vi "Pressure Regulator.vi"(7 "Indicators":T2, 8 "error in":errorcluster, 10 "Pressure Controller Port":refnum<visa-resource-name>="COM1", 11 "Controls":T1) -> (0 "error out":errorcluster)   [LabVIEW 2012, in "Pressure Regulator Controller.lvlib"]
uses:
  Pressure Regulator Controller.lvlib
  <vilib>/Instr/_visa.llb/VISA Configure Serial Port (Serial Instr).vi
panel:
  out "read buffer":string
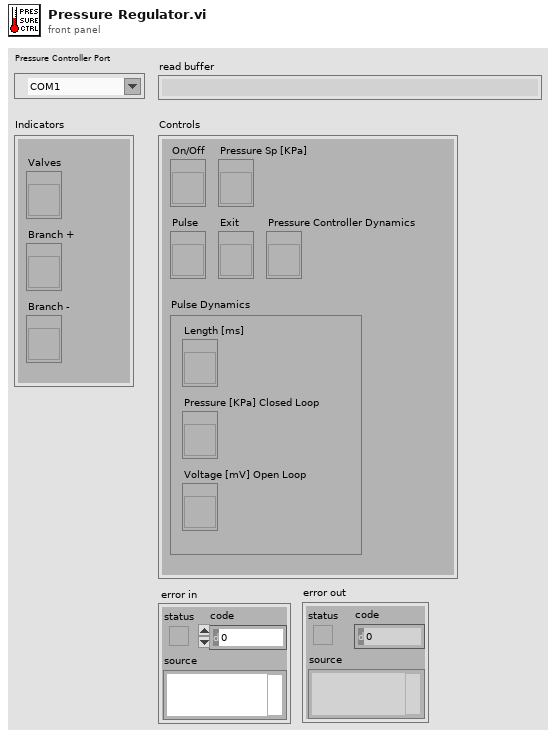
[diagram p1: front panel]
types:
  T1 = cluster{"Pulse Dynamics":cluster{"Length [ms]":refnum<vi>, "Pressure [KPa] Closed Loop":refnum<vi>, "Voltage [mV] Open Loop":refnum<vi>}, "On/Off":refnum<vi>, "Exit":refnum<vi>, "Pulse":refnum<vi>, "Pressure Sp [KPa]":refnum<vi>, "Pressure Controller Dynamics":refnum<vi>}
  T2 = cluster{"Valves":refnum<vi>, "Branch +":refnum<vi>, "Branch -":refnum<vi>}
  T3 = cluster{"Positive Branch":cluster{"Kp":dbl, "Ki":dbl, "Kd":dbl}, "Negative Branch":cluster{"Kp":dbl, "Ki":dbl, "Kd":dbl}}
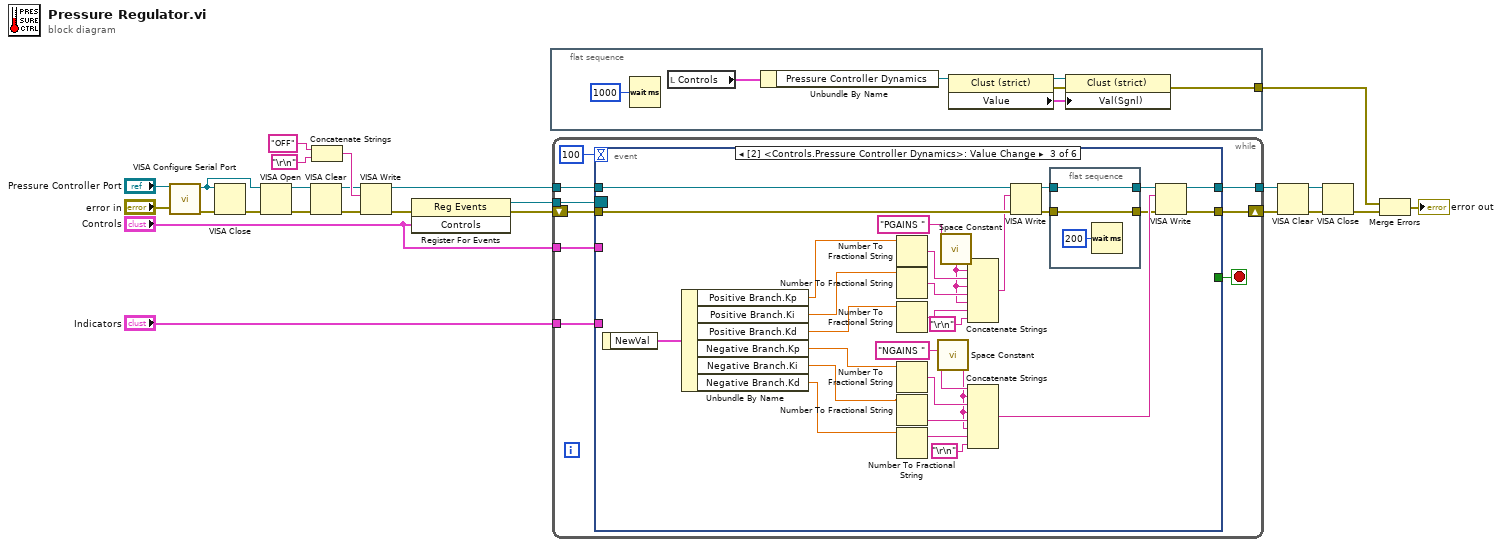
[diagram p0: block diagram]
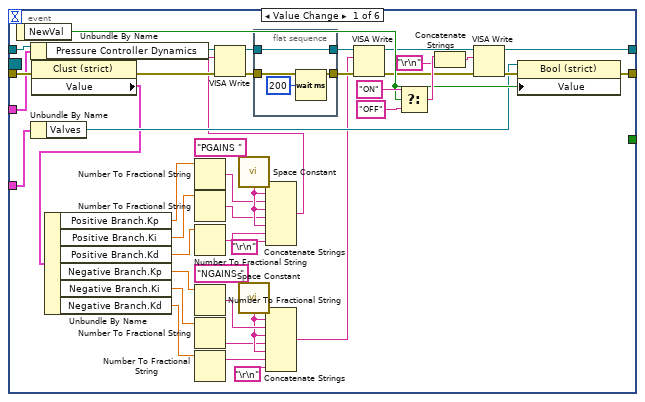
[diagram p2: hidden frame]
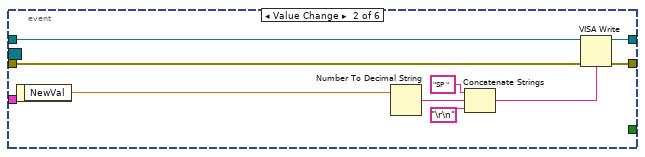
[diagram p3: hidden frame]
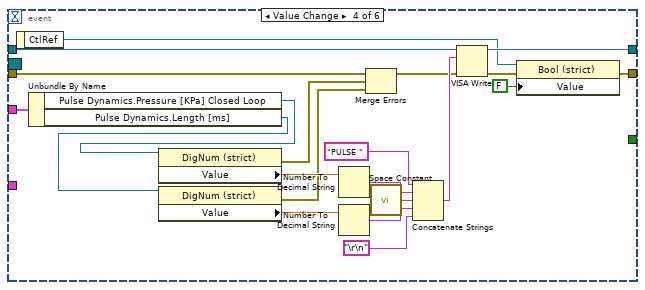
[diagram p4: hidden frame]
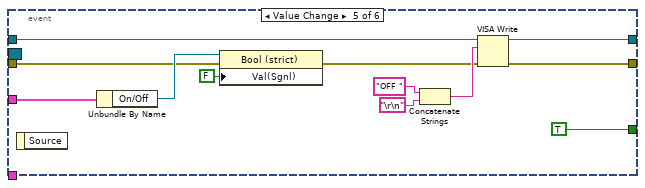
[diagram p5: hidden frame]
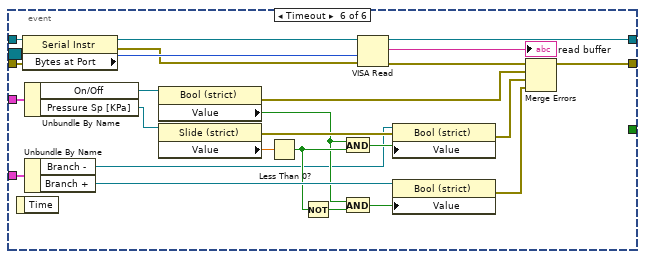
[diagram p6: hidden frame]
diagram:
  n1 = call-poly "VISA Configure Serial Port"("VISA resource name"="Pressure Controller Port", "error in (no error)"="error in") -> ("VISA resource name out"=w1:refnum<visa-resource-name>, "error out"=w3:errorcluster)  [unwired: 12 in]
  n2 = VISA Close(VISA resource name=w1, error in (no error)=w3) -> (error out=w2:errorcluster)
  n3 = VISA Open(error in (no error)=w2, VISA resource name=w1) -> (VISA resource name=w16:refnum<visa-resource-name>, error out=w17:errorcluster)  [unwired: 3 in]
  n4 = VISA Clear(VISA resource name=w16, error in (no error)=w17) -> (VISA resource name out=w10:refnum<visa-resource-name>, error out=w11:errorcluster)
  n5 = Concatenate Strings("OFF" ("string"), "\r\n") -> (w13:string)
  n6 = VISA Write(VISA resource name=w10, write buffer=w13, error in (no error)=w11) -> (VISA resource name out=w9:refnum<visa-resource-name>, error out=w12:errorcluster)  [unwired: 1 out]
  n7 = register-events(error in=w12, "Controls") -> (reference out=w19:refnum<event-registration>, error out=w21:errorcluster)  [unwired: 1 in]
  n8 = flat-sequence {
    tunnel: [w26] -> w6
    frame #0 {
      n9 = Wait (ms)(milliseconds to wait=u32 1000) -> ()  [unwired: 1 out]
      n10 = local read "Controls"() -> (w32:T1)
      n11 = Unbundle By Name(w32) -> ("Pressure Controller Dynamics"=w28:refnum<vi>)
      n12 = property class="Clust (strict)"(reference=w28) -> (reference out=w31:refnum<vi>, error out=w30:errorcluster, "Value"=w29:T3)  [unwired: 1 in]
      n13 = property class="Clust (strict)"(reference=w31, error in=w30, "Val(Sgnl)"=w29) -> (error out=w26:errorcluster)  [unwired: 1 out]
    }
  }
  n14 = while {
    tunnel: w9 -> [w33]
    shift-right: [w41] -> w23
    shift-left: w21 -> [w34]
    tunnel: [w39] -> w22
    tunnel: "Indicators" -> [w38]
    tunnel: "Controls" -> [w37]
    tunnel: w19 -> [w36]
    stop <- w35 stop-if-true
    n15 = event shown="[2] <Controls.Pressure Controller Dynamics>: Value Change" {
      selector: w36 -> [_ _ _ _ _ _]
      dyn-events: _ -> [_ _ _ _ _ _]
      timeout: 100 -> [_ _ _ _ _ _]
      tunnel: w33 -> [w46 w88 w125 w148 w159 w183]
      tunnel: [w76 w96 w118 w143 w161 w176] -> w41
      tunnel: w34 -> [w73 w89 w124 w135 w150 w181]
      tunnel: [w84 w95 w119 w149 w160 w182] -> w39
      tunnel: w38 -> [w78 _ _ _ _ w175]
      tunnel: w37 -> [w72 _ _ w140 w153 w174]
      tunnel: [_ _ _ _ TRUE _] -> w35
      event Value Change {
        n16 = event-data() -> ("NewVal"=w75:bool)  [unwired: 1 in]
        n17 = Unbundle By Name(w72) -> ("Pressure Controller Dynamics"=w71:refnum<vi>)
        n18 = Unbundle By Name(w78) -> ("Valves"=w74:refnum<vi>)
        n19 = property class="Clust (strict)"(reference=w71, error in=w73) -> (error out=w47:errorcluster, "Value"=w52:T3)  [unwired: 1 out]
        n20 = Unbundle By Name(w52) -> ("Positive Branch.Kp"=w62:dbl, "Positive Branch.Ki"=w61:dbl, "Positive Branch.Kd"=w60:dbl, "Negative Branch.Kp"=w67:dbl, "Negative Branch.Ki"=w54:dbl, "Negative Branch.Kd"=w66:dbl)
        n21 = Number To Fractional String(number=w62) -> (F-format string=w65:string)  [unwired: 3 in]
        n22 = Number To Fractional String(number=w61) -> (F-format string=w63:string)  [unwired: 3 in]
        n23 = Number To Fractional String(number=w60) -> (F-format string=w64:string)  [unwired: 3 in]
        n24 = Number To Fractional String(number=w67) -> (F-format string=w59:string)  [unwired: 3 in]
        n25 = Number To Fractional String(number=w54) -> (F-format string=w53:string)  [unwired: 3 in]
        n26 = Number To Fractional String(number=w66) -> (F-format string=w58:string)  [unwired: 3 in]
        n27 = call <vilib>:"Space Constant.vi"() -> ("String"=w69:string)
        n28 = call <vilib>:"Space Constant.vi"() -> ("String"=w56:string)
        n29 = flat-sequence {
          tunnel: [w87] -> w51
          tunnel: w50 -> [w87]
          tunnel: [w86] -> w49
          tunnel: w48 -> [w86]
          frame #0 {
            n30 = Wait (ms)(milliseconds to wait=u32 200) -> ()  [unwired: 1 out]
          }
        }
        n31 = Concatenate Strings("PGAINS " ("string"), w69, w65, w69, w63, w69, w64, "\r\n") -> (w45:string)
        n32 = VISA Write(VISA resource name=w46, write buffer=w45, error in (no error)=w47) -> (VISA resource name out=w50:refnum<visa-resource-name>, error out=w48:errorcluster)  [unwired: 1 out]
        n33 = Concatenate Strings("NGAINS " ("string"), w56, w59, w56, w53, w56, w58, "\r\n") -> (w44:string)
        n34 = VISA Write(VISA resource name=w51, write buffer=w44, error in (no error)=w49) -> (VISA resource name out=w43:refnum<visa-resource-name>, error out=w42:errorcluster)  [unwired: 1 out]
        n35 = Select(t="ON" ("string"), s=w75, f="OFF") -> (s? t:f=w80:string)
        n36 = Concatenate Strings(w80, "\r\n") -> (w83:string)
        n37 = VISA Write(VISA resource name=w43, write buffer=w83, error in (no error)=w42) -> (VISA resource name out=w84:refnum<visa-resource-name>, error out=w77:errorcluster)  [unwired: 1 out]
        n38 = property class="Bool (strict)"(reference=w74, error in=w77, "Value"=w75) -> (error out=w76:errorcluster)  [unwired: 1 out]
      }
      event Value Change {
        n39 = event-data() -> ("NewVal"=w91:dbl)  [unwired: 1 in]
        n40 = Number To Decimal String(number=w91) -> (decimal integer string=w90:string)  [unwired: 1 in]
        n41 = Concatenate Strings("SP " ("string"), w90, "\r\n") -> (w94:string)
        n42 = VISA Write(VISA resource name=w88, write buffer=w94, error in (no error)=w89) -> (VISA resource name out=w95:refnum<visa-resource-name>, error out=w96:errorcluster)  [unwired: 1 out]
      }
      event Value Change {
        n43 = event-data() -> ("NewVal"=w123:T3)  [unwired: 1 in]
        n44 = Unbundle By Name(w123) -> ("Positive Branch.Kp"=w110:dbl, "Positive Branch.Ki"=w109:dbl, "Positive Branch.Kd"=w108:dbl, "Negative Branch.Kp"=w121:dbl, "Negative Branch.Ki"=w104:dbl, "Negative Branch.Kd"=w120:dbl)
        n45 = Number To Fractional String(number=w110) -> (F-format string=w102:string)  [unwired: 3 in]
        n46 = Number To Fractional String(number=w109) -> (F-format string=w111:string)  [unwired: 3 in]
        n47 = Number To Fractional String(number=w108) -> (F-format string=w112:string)  [unwired: 3 in]
        n48 = Number To Fractional String(number=w121) -> (F-format string=w107:string)  [unwired: 3 in]
        n49 = Number To Fractional String(number=w104) -> (F-format string=w103:string)  [unwired: 3 in]
        n50 = Number To Fractional String(number=w120) -> (F-format string=w106:string)  [unwired: 3 in]
        n51 = call <vilib>:"Space Constant.vi"() -> ("String"=w98:string)
        n52 = call <vilib>:"Space Constant.vi"() -> ("String"=w101:string)
        n53 = Concatenate Strings("PGAINS " ("string"), w101, w102, w101, w111, w101, w112, "\r\n") -> (w97:string)
        n54 = Concatenate Strings("NGAINS " ("string"), w98, w107, w98, w103, w98, w106, "\r\n") -> (w117:string)
        n55 = VISA Write(VISA resource name=w125, write buffer=w97, error in (no error)=w124) -> (VISA resource name out=w115:refnum<visa-resource-name>, error out=w113:errorcluster)  [unwired: 1 out]
        n56 = flat-sequence {
          tunnel: [w128] -> w116
          tunnel: w115 -> [w128]
          tunnel: [w127] -> w114
          tunnel: w113 -> [w127]
          frame #0 {
            n57 = Wait (ms)(milliseconds to wait=u32 200) -> ()  [unwired: 1 out]
          }
        }
        n58 = VISA Write(VISA resource name=w116, write buffer=w117, error in (no error)=w114) -> (VISA resource name out=w119:refnum<visa-resource-name>, error out=w118:errorcluster)  [unwired: 1 out]
      }
      event Value Change {
        n59 = event-data() -> ("CtlRef"=w142:refnum<vi>)  [unwired: 1 in]
        n60 = Unbundle By Name(w140) -> ("Pulse Dynamics.Pressure [KPa] Closed Loop"=w139:refnum<vi>, "Pulse Dynamics.Length [ms]"=w138:refnum<vi>)
        n61 = property class="DigNum (strict)"(reference=w139) -> (error out=w133:errorcluster, "Value"=w137:dbl)  [unwired: 1 in, 1 out]
        n62 = property class="DigNum (strict)"(reference=w138) -> (error out=w132:errorcluster, "Value"=w136:dbl)  [unwired: 1 in, 1 out]
        n63 = Number To Decimal String(number=w137) -> (decimal integer string=w145:string)  [unwired: 1 in]
        n64 = Number To Decimal String(number=w136) -> (decimal integer string=w131:string)  [unwired: 1 in]
        n65 = Merge Errors(w135, w133, w132) -> (w134:errorcluster)
        n66 = call <vilib>:"Space Constant.vi"() -> ("String"=w129:string)
        n67 = Concatenate Strings("PULSE " ("string"), w145, w129, w131, "\r\n") -> (w147:string)
        n68 = VISA Write(VISA resource name=w148, write buffer=w147, error in (no error)=w134) -> (VISA resource name out=w149:refnum<visa-resource-name>, error out=w144:errorcluster)  [unwired: 1 out]
        n69 = property class="Bool (strict)"(reference=w142, error in=w144, "Value"=FALSE) -> (error out=w143:errorcluster)  [unwired: 1 out]
      }
      event Value Change {
        n70 = event-data() -> ()  [unwired: 1 in, 1 out]
        n71 = Unbundle By Name(w153) -> ("On/Off"=w152:refnum<vi>)
        n72 = property class="Bool (strict)"(reference=w152, error in=w150, "Val(Sgnl)"=FALSE ("Value")) -> (error out=w151:errorcluster)  [unwired: 1 out]
        n73 = Concatenate Strings("OFF " ("string"), "\r\n") -> (w158:string)
        n74 = VISA Write(VISA resource name=w159, write buffer=w158, error in (no error)=w151) -> (VISA resource name out=w160:refnum<visa-resource-name>, error out=w161:errorcluster)  [unwired: 1 out]
      }
      event Timeout {
        n75 = event-data() -> ()  [unwired: 1 in, 1 out]
        n76 = property class="Serial Instr"(reference=w183, error in=w181) -> (reference out=w186:refnum<visa-resource-name>, error out=w184:errorcluster, "Bytes at Port"=w185:u32)
        n77 = Unbundle By Name(w174) -> ("On/Off"=w171:refnum<vi>, "Pressure Sp [KPa]"=w172:refnum<vi>)
        n78 = Unbundle By Name(w175) -> ("Branch -"=w165:refnum<vi>, "Branch +"=w177:refnum<vi>)
        n79 = property class="Bool (strict)"(reference=w171) -> (error out=w164:errorcluster, "Value"=w167:bool)  [unwired: 1 in, 1 out]
        n80 = property class="Slide (strict)"(reference=w172) -> (error out=w169:errorcluster, "Value"=w170:dbl)  [unwired: 1 in, 1 out]
        n81 = Less Than 0?(x=w170) -> (x < 0?=w168:bool)
        n82 = Not(x=w168) -> (.not. x?=w166:bool)
        n83 = And(x=w167, y=w168) -> (x .and. y?=w178:bool)
        n84 = And(x=w167, y=w166) -> (x .and. y?=w179:bool)
        n85 = VISA Read(VISA resource name=w186, byte count=w185, error in (no error)=w184) -> (VISA resource name out=w182:refnum<visa-resource-name>, read buffer=→"read buffer":string, error out=w173:errorcluster)  [unwired: 1 out]
        n86 = property class="Bool (strict)"(reference=w165, error in=w169, "Value"=w178) -> (error out=w163:errorcluster)  [unwired: 1 out]
        n87 = property class="Bool (strict)"(reference=w177, "Value"=w179) -> (error out=w162:errorcluster)  [unwired: 1 in, 1 out]
        n88 = Merge Errors(w173, w164, w163, w162) -> (w176:errorcluster)
      }
    }
  }
  n89 = VISA Clear(VISA resource name=w22, error in (no error)=w23) -> (VISA resource name out=w25:refnum<visa-resource-name>, error out=w24:errorcluster)
  n90 = VISA Close(VISA resource name=w25, error in (no error)=w24) -> (error out=w5:errorcluster)
  n91 = Merge Errors(w6, w5) -> (→"error out":errorcluster)
